vi "core_error_if_not_cluster.vi"(8 "Error in":errorcluster caption="Error in (no error)", 11 "Cluster":variant) -> (0 "Error out":errorcluster, 3 "Cluster duplicate":variant)   [LabVIEW 2015]
uses:
  <vilib>/Utility/Data Type/Type Definitions/Data Type.ctl
  <vilib>/Utility/Data Type/NI_Data Type.lvlib
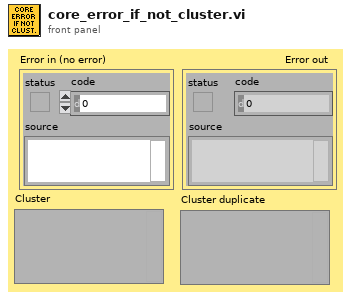
[diagram p1: front panel]
types:
  T1 = typedef "NI_Data Type.lvlib/Data Type.ctl" = enum8{"Invalid Type", "Void", "I8", "I16", "I32", "I64", "U8", "U16", "U32", "U64", "Single Float", "Double Float", "Extended Float", "Single Complex", "Double Complex", "Extended Complex", "Enum U8", "Enum U16", "Enum U32", "Enum U64", "Single Float With Unit", "Double Float With Unit", "Extended Float With Unit", "Single Complex with Unit", "Double Complex with Unit", "Extended Complex with Unit", "Boolean", "String", "Path", "Picture", "Tag", "Array", "Cluster", "Variant", "LV Variant", "Waveform", "Timestamp", "Digital Waveform", "Digital Data", "ExpressData", "Refnum", "External Data", "VI", "Poly VI", "LabVIEW Class Instance", "Fixed Point"}
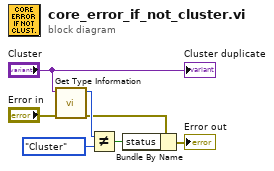
[diagram p0: block diagram]
diagram:
  n1 = call <vilib>:"Get Type Information.vi"("error in (no error)"="Error in", "Variant"="Cluster") -> ("error out"=w1:errorcluster, "Type"=w4:T1)  [unwired: 5 in, 3 out]
  n2 = Not Equal?(x=w4, y=Data_Type."Cluster" ("Type")) -> (x != y?=w6:bool)
  n3 = Bundle By Name(cluster=w1, "status"=w6) -> (→"Error out":errorcluster)
  "Cluster duplicate" <- "Cluster"
